vi "Register Descriptors.vi"(8 "error in (no error)":errorcluster, 11 "gRPC ID":T1) -> (0 "error out":errorcluster, 3 "gRPC ID Out":T1)   [LabVIEW 2021, in "CIF_Manager_server.lvlib"]
uses:
  CIF_Manager_server.lvlib
  <vilib>/gRPC/LabVIEW gRPC Library/Shared/grpcId.ctl
  <vilib>/gRPC/LabVIEW gRPC Library/grpc-lvsupport-release.lvlib
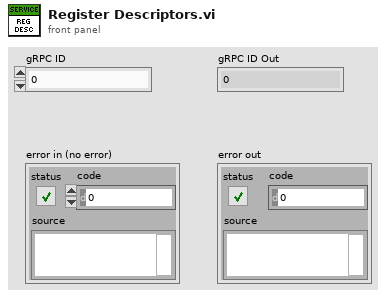
[diagram p1: front panel]
types:
  T1 = typedef "grpc-lvsupport-release.lvlib/grpcId.ctl" = u64
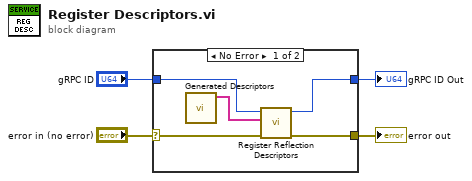
[diagram p0: block diagram]
diagram:
  n1 = case shown="No Error" "error in (no error)" {
    selector: "error in (no error)" -> [w9 w11]
    tunnel: [w6 w10] -> w1
    tunnel: [w8 w11] -> w4
    tunnel: "gRPC ID" -> [w5 w10]
    frame No Error {
      n2 = call "Generated Descriptors.vi"() -> ("Descriptor Strings"=w7:string[])  [unwired: 11 in]
      n3 = call <vilib>:"Register Reflection Descriptors.vi"("error in"=w9, "reflector description strings"=w7, "gRPCid in"=w5) -> ("error out"=w8:errorcluster, "gRPCid out"=w6:T1)  [unwired: 7 in]
    }
    frame Error {
    }
  }
  "error out" <- w4
  "gRPC ID Out" <- w1
